vi "Create.vi"(8 "error in (no error)":errorcluster, 9 "launcher_name":string, 10 "pid":u32, 11 "Plugin Manager in":refnum<class "CIFLauncher.lvclass">) -> (0 "error out":errorcluster, 3 "Plugin Manager out":refnum<class "CIFLauncher.lvclass">)   [LabVIEW 2021, in "CIFLauncher.lvclass"]
uses:
  CIFLauncher.lvclass
  CIFUtilities/CIFLogs/Typedef/Message Type.ctl
  typedef/Loaded Plugin Map.ctl
  CIFLauncher.lvclass/CIFLauncher.ctl
  CIFUtilities/CIFConfigurationFile/CIF Configuration File.lvlib
  CIFUtilities/CIFLogs/CIFLogs.lvlib
  gRPC/CIF_Launcher_server/RPC Messages/cif_manager_LauncherType.ctl
  gRPC/CIF_Launcher_server/CIF_Launcher_server.lvlib
  CIFPluginManager/gRPC/CIF_Manager_Client_Wrapper/CIFManagerClientWrapper.lvlib
  CIFPluginManager/gRPC/CIF_Manager_client/RPC Messages/cif_manager_LauncherType.ctl
  CIFPluginManager/gRPC/CIF_Manager_client/CIF_Manager_client.lvlib
  CIFPluginManager/gRPC/CIF_Manager_client/RPC Messages/cif_manager_LauncherInfo.ctl
  CIFPluginManager/gRPC/CIF_Manager_client/RPC Messages/cif_common_Status.ctl
  CIFPluginManager/gRPC/CIF_Manager_client/RPC Messages/cif_manager_LauncherStatus.ctl
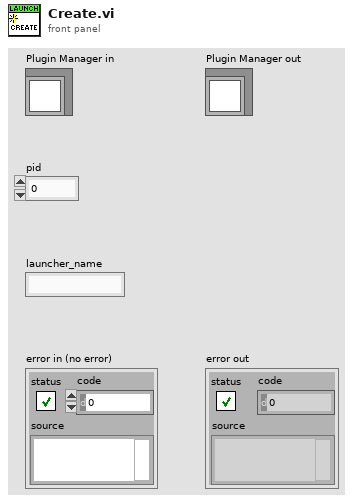
[diagram p1: front panel]
types:
  T1 = typedef "CIF_Manager_client.lvlib/cif_manager_LauncherStatus.ctl" = cluster{"launcher_info":T2, "grpc_port":i32, "pid":u32, "status":T4}
  T2 = typedef "CIF_Manager_client.lvlib/cif_manager_LauncherInfo.ctl" = cluster{"launcher_type":T3, "launcher_name":string}
  T3 = typedef "CIF_Manager_client.lvlib/cif_manager_LauncherType.ctl" = enum32{"LAUNCHERTYPE_UNKNOWN", "LAUNCHERTYPE_LABVIEW"}
  T4 = typedef "CIF_Manager_client.lvlib/cif_common_Status.ctl" = cluster{"code":i32, "message":string}
  T5 = typedef "CIF_Launcher_server.lvlib/cif_manager_LauncherType.ctl" = enum32{"LAUNCHERTYPE_UNKNOWN", "LAUNCHERTYPE_LABVIEW"}
  T6 = typedef "CIFLauncher.lvclass/Loaded Plugin Map.ctl" = map{string, refnum<vi>}
  T7 = typedef "CIFLogs.lvlib/Message Type.ctl" = enum16{"Error", "Information", "Print Terminal", "Configuration"}
  T8 = typedef "CIF_Launcher_server.lvlib/cif_manager_LauncherInfo.ctl" = cluster{"launcher_type":T5, "launcher_name":string}
  T9 = typedef "grpc-lvsupport-release.lvlib/grpcId.ctl" = u64
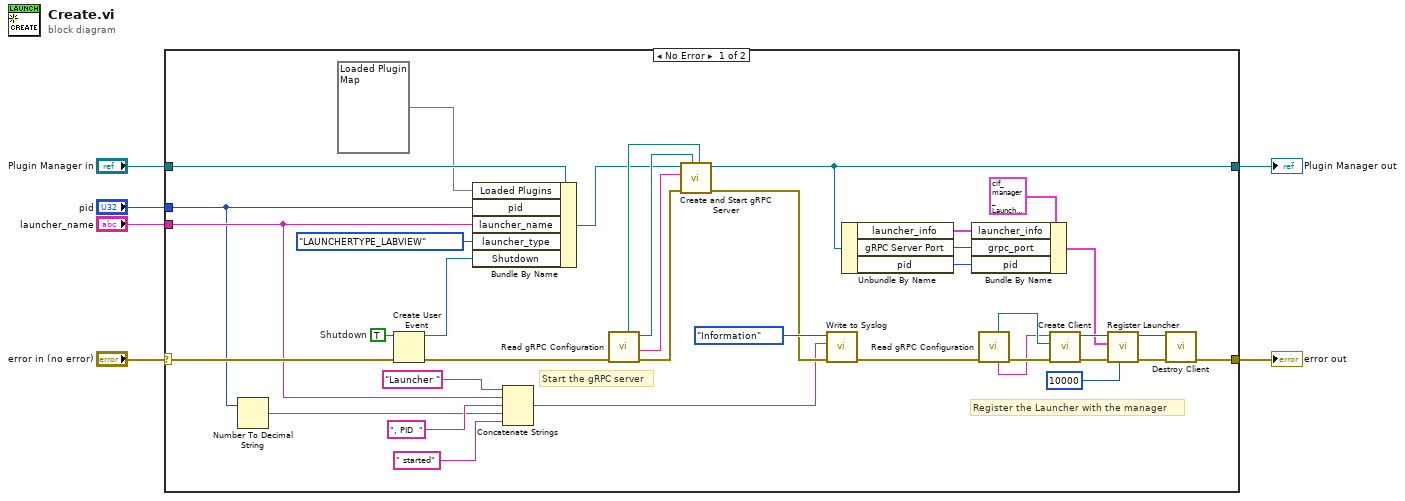
[diagram p0: block diagram]
diagram:
  n1 = case shown="No Error" "error in (no error)" {
    selector: "error in (no error)" -> [w37 w45]
    tunnel: [w18 w45] -> w5
    tunnel: [w11 w44] -> w3
    tunnel: "Plugin Manager in" -> [w34 w44]
    tunnel: "pid" -> [w24 _]
    tunnel: "launcher_name" -> [w28 _]
    frame No Error {
      w38 = TRUE  # Shutdown
      # "Register the Launcher with the manager"
      # "Start the gRPC server"
      n2 = Number To Decimal String(number=w24) -> (decimal integer string=w23:string)  [unwired: 1 in]
      n3 = Create User Event(user event datatype=w38, error in=w37) -> (user event=w31:refnum<user-event>, error out=w36:errorcluster)
      n4 = Bundle By Name(cluster=w34, "Loaded Plugins"=T6 {}, "pid"=w24, "launcher_name"=w28, "launcher_type"=cif_manager_LauncherType."LAUNCHERTYPE_LABVIEW" ("launcher_info.launcher_type"), "Shutdown"=w31) -> (w30:refnum<class "CIFLauncher.lvclass">)
      n5 = Concatenate Strings("Launcher " ("message"), w28, ", PID  " ("message"), w23, " started" ("message")) -> (w25:string)
      n6 = call "Read gRPC Configuration.vi"("error in"=w36) -> ("error out"=w43:errorcluster, "Manager Server Address"=w40:string, "Server Certificate File (.crt)"=w41:path, "Server Key File (.key)"=w42:path)  [unwired: 5 in, 2 out]
      n7 = call "Create and Start gRPC Server.vi"("Server Key File (.key)"=w42, "Server Certificate File (.crt)"=w41, "error in (no error)"=w43, "Server Address"=w40, "CIFLauncher in"=w30) -> ("error out"=w35:errorcluster, "CIFLauncher out"=w11:refnum<class "CIFLauncher.lvclass">)  [unwired: 5 in]
      n8 = call "Write to Syslog.vi"("error in (no error)"=w35, "message"=w25, "CIF Message Type"=Message_Type."Information") -> ("error out"=w17:errorcluster)  [unwired: 8 in]
      n9 = Unbundle By Name(w11) -> ("launcher_info"=w10:T8, "gRPC Server Port"=w9:i32, "pid"=w8:u32)
      n10 = Bundle By Name(cluster=T1 {"launcher_info"={"launcher_type"=enum."LAUNCHERTYPE_UNKNOWN", "launcher_name"=""}, "grpc_port"=0, "pid"=0, "status"={"code"=0, "message"=""}} ("Launcher"), "launcher_info"=w10, "grpc_port"=w9, "pid"=w8) -> (w7:T1)
      n11 = call "Read gRPC Configuration.vi"("error in"=w17) -> ("error out"=w16:errorcluster, "Local Manager Address"=w14:string, "Server Key File (.key)"=w15:path)  [unwired: 5 in, 3 out]
      n12 = call "Create Client.vi"("error in"=w16, "Server Certificate File (.crt)"=w15, "address"=w14) -> ("error out"=w21:errorcluster, "gRPC ID Out"=w22:T9)  [unwired: 7 in]
      n13 = call "Register Launcher.vi"("timeout (ms)"=10000, "error in"=w21, "Launcher"=w7, "gRPC ID in"=w22) -> ("error out"=w19:errorcluster, "gRPC ID out"=w20:T9)  [unwired: 6 in]
      n14 = call "Destroy Client.vi"("error in"=w19, "gRPC ID"=w20) -> ("error out"=w18:errorcluster)  [unwired: 9 in]
    }
    frame Error {
    }
  }
  "error out" <- w5
  "Plugin Manager out" <- w3
